vi "FPGAController_v5.vi"() -> ()   [LabVIEW 2015]
uses:
  <vilib>/Utility/miscctls.llb/LVPointTypeDef.ctl
  <vilib>/FPGAPlugInAG/PXIe-7971R/niLvFpga_Open_PXIe-7971R.vi
  <userlib>/_OpenG.lib/comparison/comparison.llb/DBL Changed__ogtk.vi
  <userlib>/_OpenG.lib/file/file.llb/Strip Path Extension - Path__ogtk.vi
  <userlib>/_OpenG.lib/comparison/comparison.llb/Boolean Changed__ogtk.vi
  <vilib>/Utility/error.llb/Error Cluster From Error Code.vi
  <vilib>/rvi/errors/niLvFpgaAdjustHostInterfaceError.vi
  <vilib>/addons/database/Connection.llb/Conn Execute.vi
  <vilib>/addons/database/Recordset.llb/Rec Fetch Recordset Data (R).vi
  <vilib>/addons/database/Recordset.llb/Rec Destroy - Connection.vi
  <vilib>/FPGAPlugInAG/PXIe-7971R/niLvFpga_Close_PXIe-7971R.vi
  <vilib>/rvi/interface/nirviOpenFPGA/nirviOpenFPGA.xnode
  FPGA Bitfiles/FPGA2_FPGATarget_FPGAcode2_Gw4Ab0yitnw.lvbitx
  <vilib>/rvi/interface/nirviMethod/nirviMethod.xnode
  <vilib>/FPGA/interface/niFpgaViExecutionMode.ctl
  <vilib>/rvi/interface/nirviReadWriteControl/nirviReadWriteControl.xnode
  <vilib>/addons/database/_DB Variant To Data/Database Variant To Data.xnode
  <vilib>/rvi/interface/nirviCloseFPGA/nirviCloseFPGA.xnode
  <vilib>/addons/database/NI_Database_API.lvlib
  NiFpgaLv.dll
panel:
  out "Time Betwee Shots":dbl
  out "Del Armed":bool
  in  "Lower Threshold":bool
  in  "Raise Threshold":bool
  out "Update Threshold":bool
  in  "Min. Time\nBetween Shots (s)":dbl
  in  "Rate Limiting":bool
  out "Armed":bool
  in  "Add Delay":bool
  in  "Delay Name":string
  in  "Delay Value":dbl=3.0 min=0.0
  in  "Delay Ring":dbl(ring)=3.15039 items=["Ablation Chamber"=6.45, "LEIL Chamber"=4.318, "Third Detector"=3.15039, "Custom"=0.0]
  in  "Rearm Trigger":bool
  in  "One Shot Mode":bool
  out "Last Update:":timestamp
  out "Updating FPGA":bool
  out "Sensitivity":dbl
  out "error out":errorcluster
  out "Low Mass Limit":fxp<+,31,17>
  out "High Mass Limit":fxp<+,31,17>
  out "stopping":bool
  in  "Auto Threshold":bool
  out "Peletron (MV)":dbl=2.0
  out "High Mass (kg)":dbl=inf
  out "Low Mass (kg)":dbl
  out "High Charge Limit":i16
  out "Low Charge Limit":i16
  out "High velocity count":i32=210
  out "Low velocity count":i32=21000
  in  "stop":bool
  in  "Peak-Threshold Factor":dbl=2.0
  out "Low Charge Limit (fC)":dbl
  out "High Charge Limit (fC)":dbl=100.0
  out "High Velocity":dbl=100000.0
  out "Low Velocity":dbl=1000.0
  out "Filter 7 Peak":i32=7483
  out "Filter 6 Peak":i32=9863
  out "Filter 5 Peak":i32=13910
  out "Filter 4 Peak":i32=18191
  out "Filter 3 Peak":i32=46254
  out "Filter 2 Peak":i32=120664
  out "Filter 1 Peak":i32=295996
  in  "Filter7 Threshold":i32=-21165
  in  "Filter6 Threshold":i32=-29358
  in  "Filter5 Threshold":i32=-41730
  in  "Filter4 Threshold":i32=-54306
  in  "Filter3 Threshold":i32=-138762
  in  "Filter2 Threshold":i32=-361992
  in  "Filter1 Threshold":i32=-887988
  in  "Zero Peak Values":bool
  in  "Assign Threshold":bool
  in  "Run Mode":bool
  # "Settings"
  # "Dubugging"
  # "Independent Variable"
  # "Low Vel."
  # "High Vel."
  # "Low Q (fC)"
  # "High Q (fC)"
  # "Plate Control While Loop Counter"
  # "Low Mass (kg)"
  # "High Mass (kg)"
  # "Sens. (V/pC)"
  # "Peletron (MV)"
  # "Current Value of Running Average"
  # "Peak Threshold Factor"
  # "Delay Trigger"
  # "Dist. from 2nd Det. (m)"
  # "Name"
  # "Peak Values"
  # "Peak 1"
  # "Peak 2"
  # "Peak 3"
  # "Peak 4"
  # "Peak 5"
  # "Peak 6"
  # "Peak 7"
  # "Thresholds"
  # "Threshold 1"
  # "Threshold 2"
  # "Threshold 3"
  # "Threshold 4"
  # "Threshold 5"
  # "Threshold 6"
  # "Threshold 7"
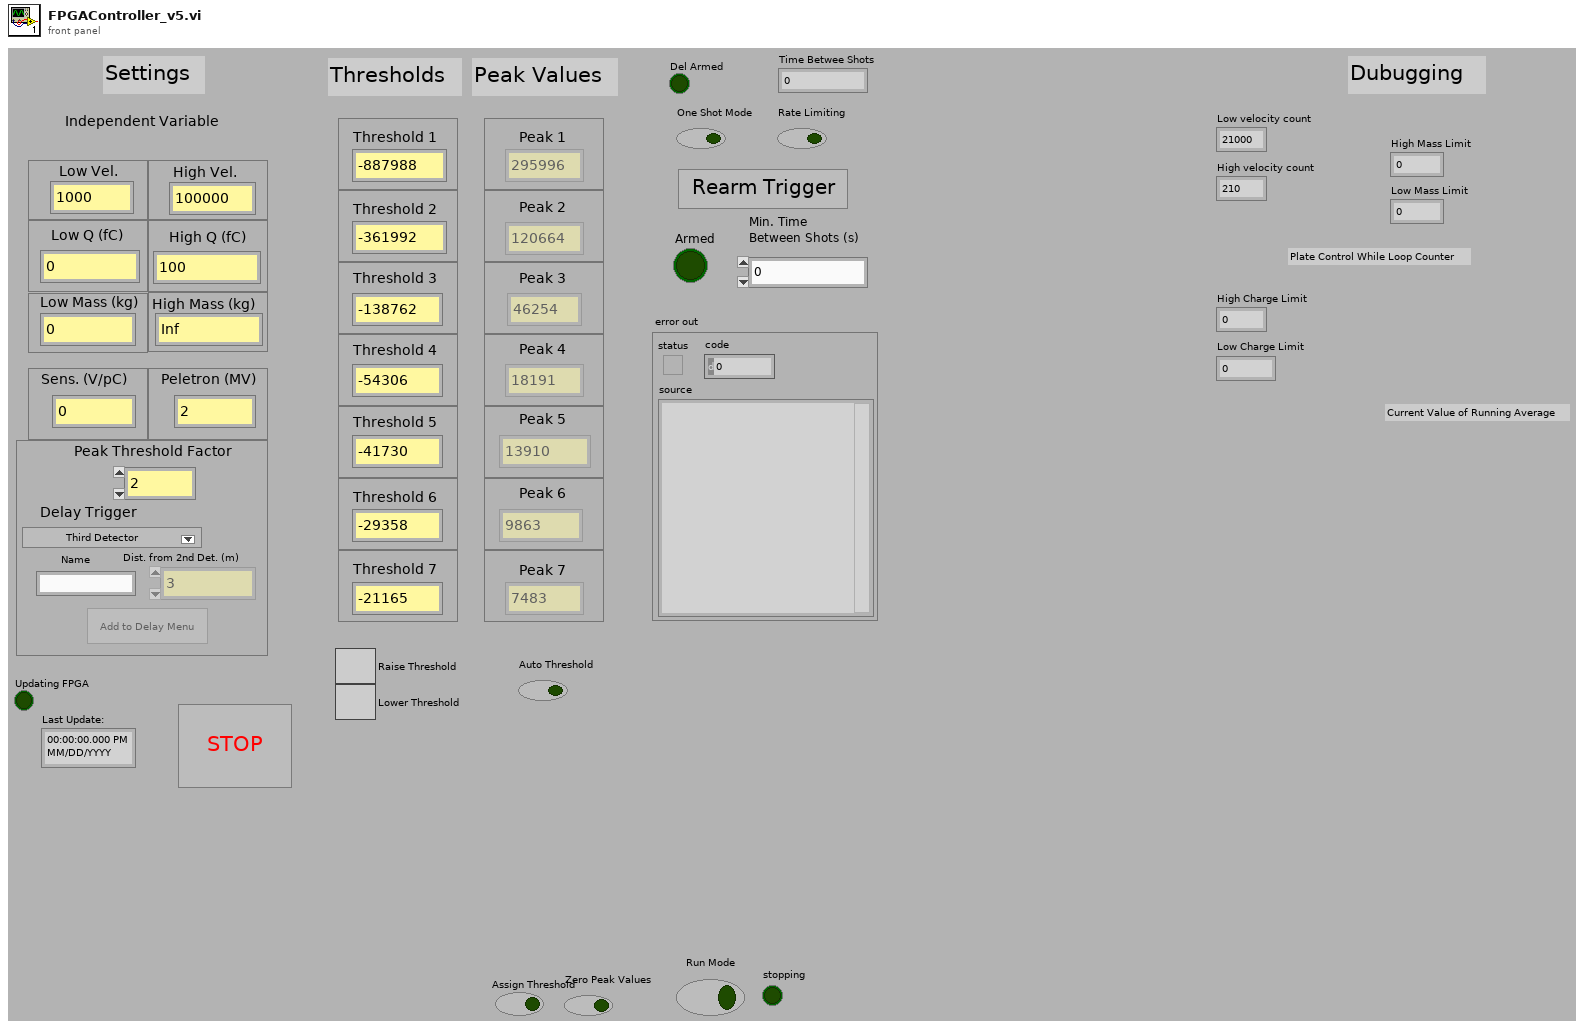
[diagram p1: front panel]
types:
  T1 = typedef "LVPointTypeDef.ctl" = cluster{"Horizontal":i16, "Vertical":i16}
  T2 = enum8{"Enabled", "Disabled", "Disabled and Grayed Out"}
  T3 = typedef "NI_Database_API.lvlib/Conn ObjectReference.ctl" = refnum<k1>
  T4 = cluster{"Filter 1 Peak":i32, "Filter 2 Peak":i32, "Filter 3 Peak":i32, "Filter 4 Peak":i32, "Filter 5 Peak":i32, "Filter 6 Peak":i32, "Filter 7 Peak":i32}
  T5 = typedef "NI_Database_API.lvlib/Rec ObjectReference.ctl" = refnum<k1>
  T6 = cluster{"Numeric":dbl, "Numeric":dbl, "Numeric":dbl, "Numeric":dbl, "Numeric":dbl, "Numeric":dbl, dbl, dbl, "Value":dbl, fxp<+,16,7>, bool}
  T7 = typedef "LVStringsAndValuesArrayTypeDef_DBL.ctl" = cluster{"String":string, "Value":dbl}[]
  T8 = cluster{"Low Velocity Count":i32, "High Velocity Count":i32, "Low Charge Limit (ADC ticks)":i16, "High Charge Limit (ADC ticks)":i16, "Low Mass (ADC*cycle^2)":i64, "High Mass (ADC*cycle^2)":i64, "Mult":fxp<+,16,7>, "Mult Use?":bool}
  T9 = cluster{"Detector 3 Correlation 1":i16, "Detector 3 Correlation 2":i16, "Detector 3 Correlation 3":i16, "Detector 3 Correlation 4":i16, "Detector 3 Correlation 5":i16, "Detector 3 Correlation 6":i16, "Detector 3 Correlation 7":i16}
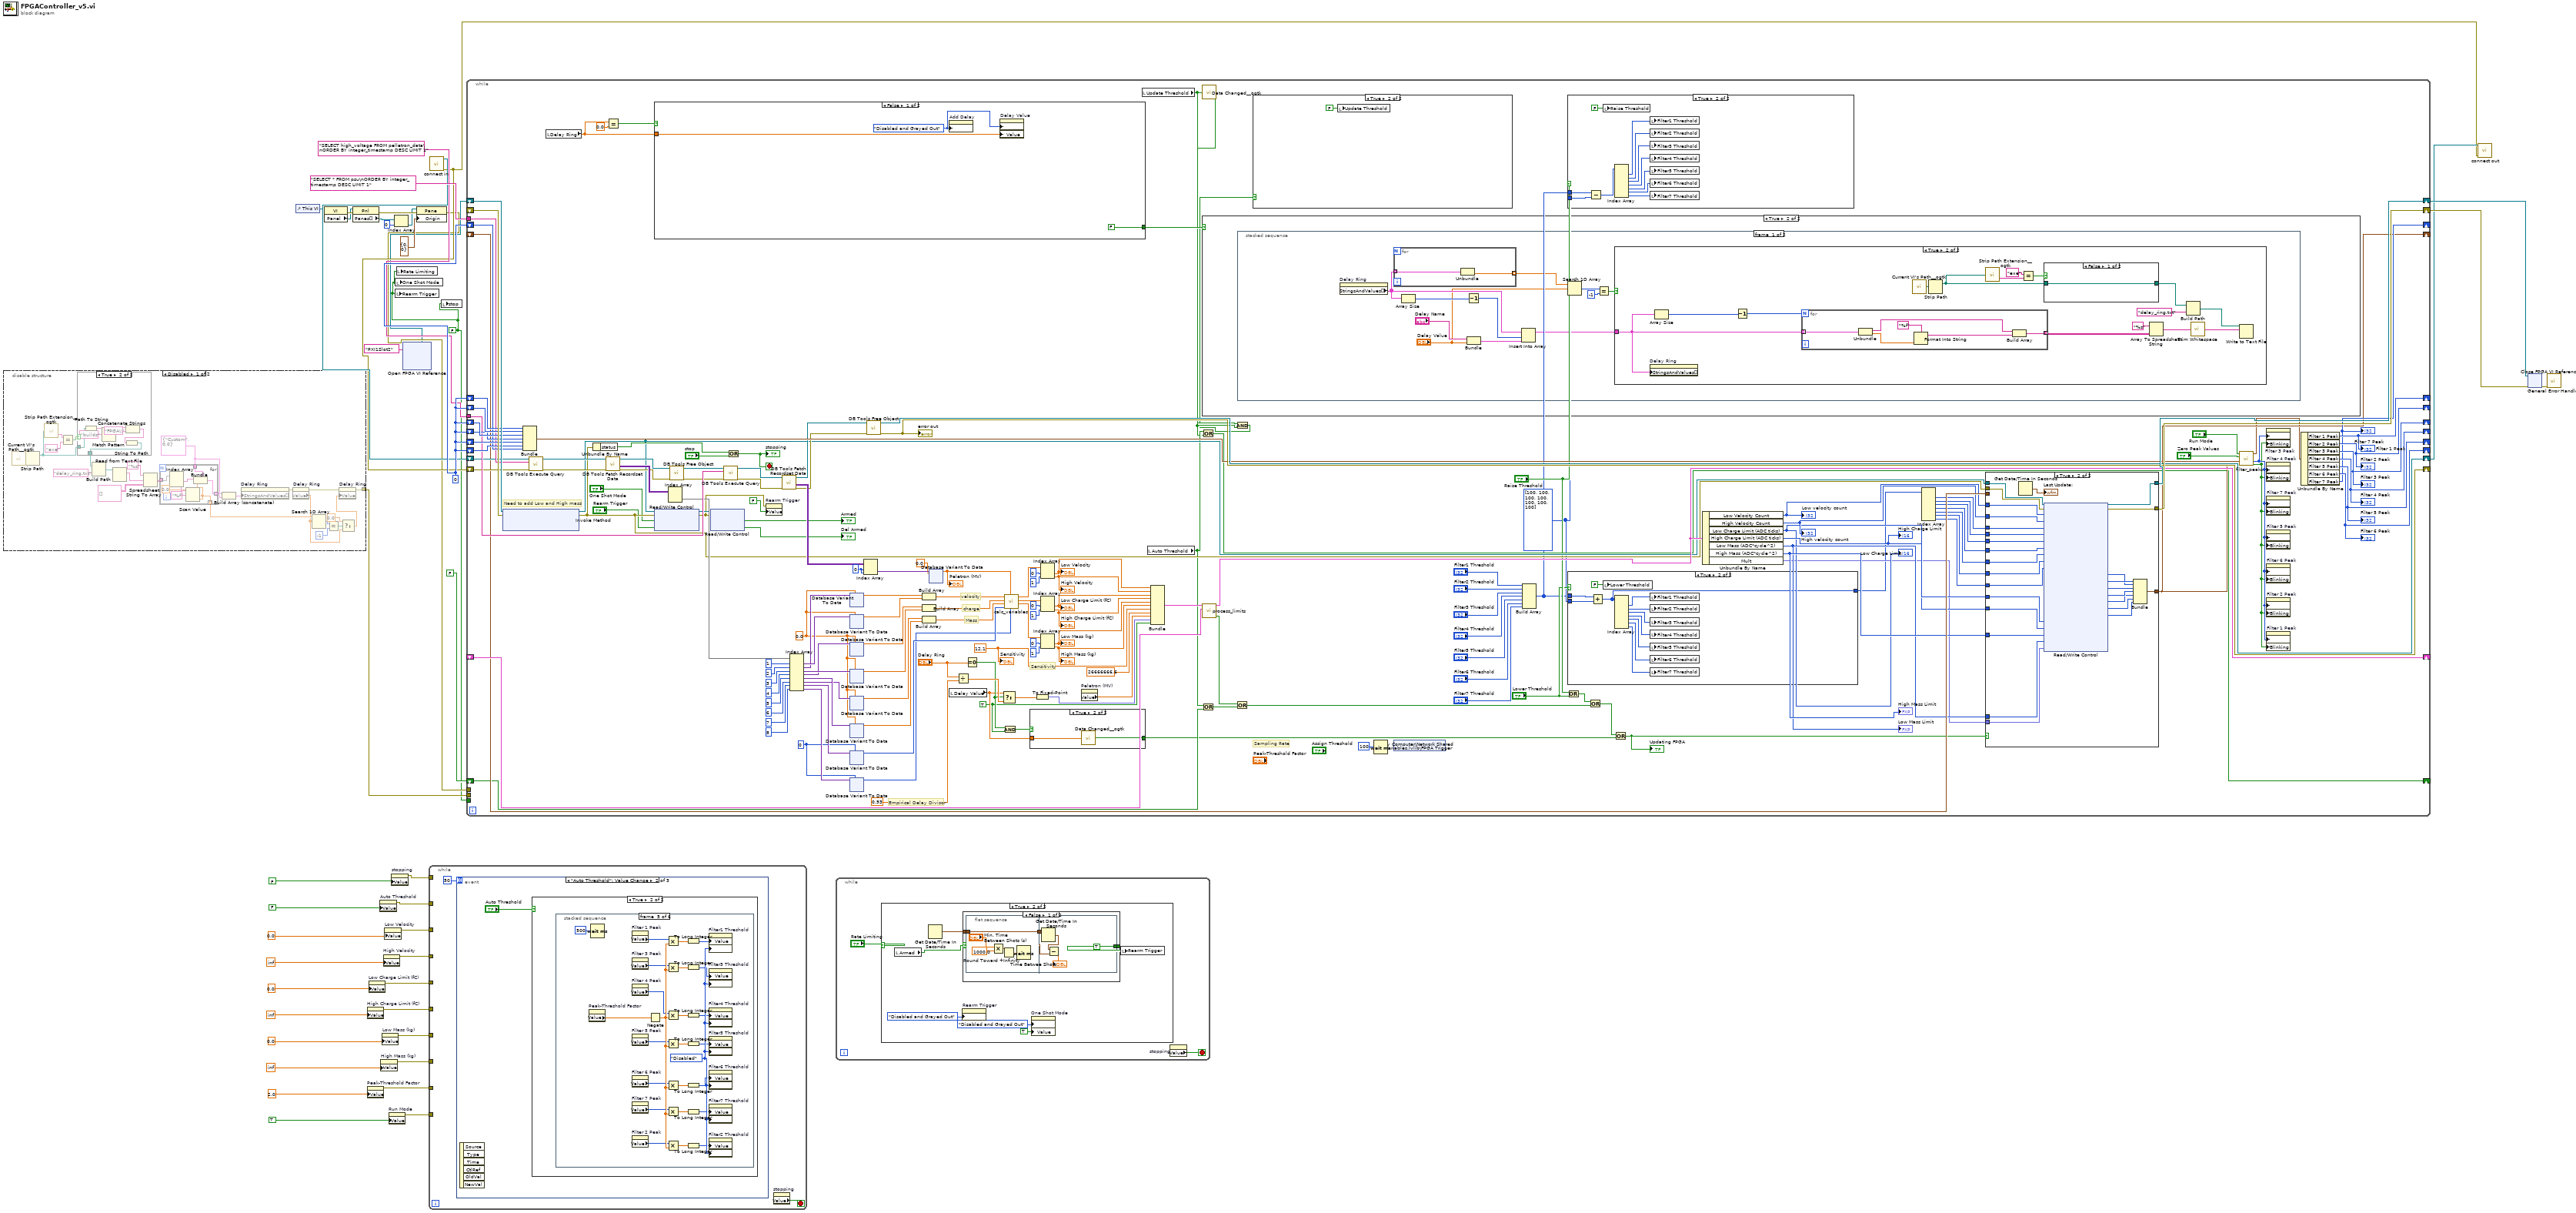
[diagram p0: block diagram]
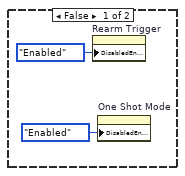
[diagram p4: hidden frame]
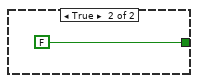
[diagram p5: hidden frame]
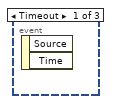
[diagram p6: hidden frame]
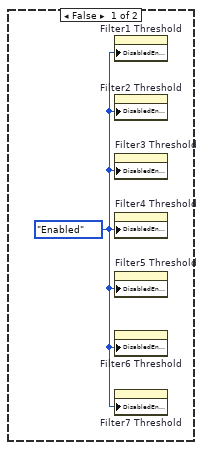
[diagram p7: hidden frame]
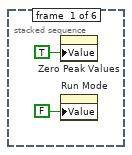
[diagram p8: hidden frame]
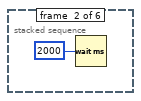
[diagram p9: hidden frame]
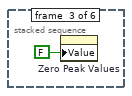
[diagram p10: hidden frame]
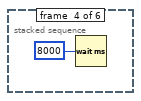
[diagram p11: hidden frame]
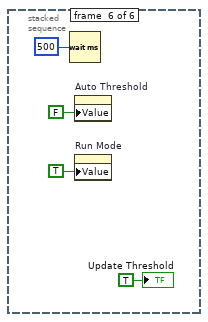
[diagram p12: hidden frame]
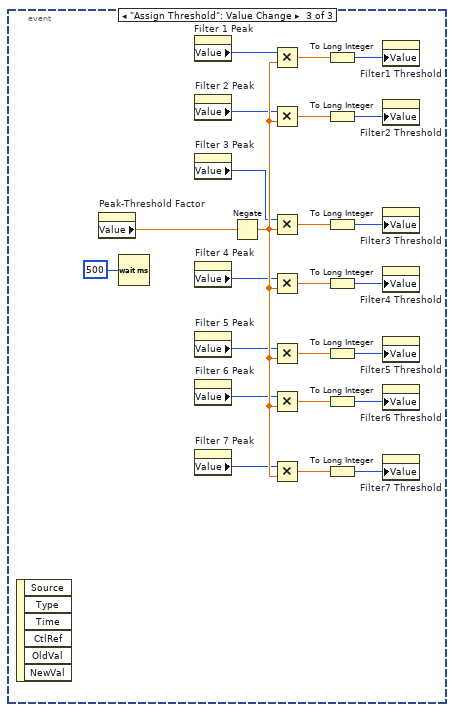
[diagram p13: hidden frame]
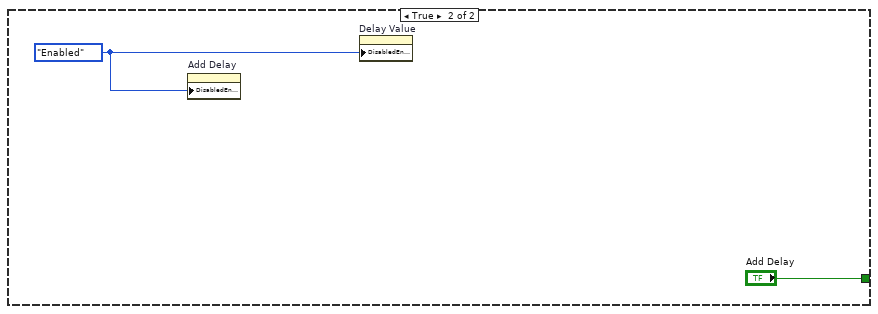
[diagram p18: hidden frame]
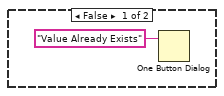
[diagram p20: hidden frame]
diagram:
  w1 = FALSE
  w42 = 0
  n1 = disable-structure shown="Disabled" {
    disable-tunnel: [w50 _] -> w3
    frame Disabled {
      w59 = cluster{"String":string, "Value":dbl} {"String"="Custom", "Value"=0.0}
      n2 = call <userlib>:"Current VI's Path__ogtk.vi"() -> ("Current VI's Path (+ Relative)"=w68:path)  [unwired: 1 in]
      n3 = Strip Path(path=w68) -> (stripped path=w54:path)  [unwired: 1 out]
      n4 = call-poly <userlib>:"Strip Path Extension__ogtk.vi"("path"=w54) -> ("extension"=w58:string)  [unwired: 1 out]
      n5 = Equal?(x=w58, y="exe") -> (x = y?=w55:bool)
      n6 = case shown="True" w55 {
        tunnel: w54 -> [w77 w84]
        tunnel: [w77 w78] -> w53
        frame False {
        }
        frame True {
          n7 = Path To String(path=w84) -> (string=w83:string)
          n8 = Match Pattern(string=w83, regular expression="builds") -> (before substring=w81:string)  [unwired: 1 in, 3 out]
          n9 = Concatenate Strings(w81, "FPGA\\" ("string")) -> (w79:string)
          n10 = String To Path(string=w79) -> (path=w78:path)
        }
      }
      n11 = Build Path(base path=w53, name or relative path="delay_ring.txt") -> (appended path=w56:path)
      n12 = Read from Text File(file (use dialog)=w56) -> (text=w66:string)  [unwired: 3 in, 3 out]
      n13 = Spreadsheet String To Array(format string="%s", spreadsheet string=w66, array type (2D Dbl)=string[][] []) -> (array=w63:string[][])  [unwired: 1 in]
      n14 = for {
        tunnel: w63 -> [w76] mode=indexing
        tunnel: w59 -> [w74]
        tunnel: [w70] -> w60 mode=indexing
        tunnel: [w69] -> w52 mode=indexing
        n15 = Index Array(array=w76) -> (element #1=w75:string, element #2=w73:string)  [unwired: 2 in]
        n16 = Scan Value(string=w73, format string="%f", default (0 dbl)=0.0) -> (value=w69:dbl)  [unwired: 1 out]
        n17 = Bundle(cluster=w74, "String"=w75, "Value"=w69) -> (w70:cluster{"String":string, "Value":dbl})
      }
      n18 = Build Array (concatenate)(w60, w59) -> (w62:cluster{"String":string, "Value":dbl}[])
      n19 = property on="Delay Ring" class="Ring (strict)"("StringsAndValues[]"=w62) -> (error out=w61:errorcluster)  [unwired: 2 in, 1 out]
      n20 = property on="Delay Ring" class="Ring (strict)"(error in=w61) -> (error out=w51:errorcluster, "Value"=w45:dbl)  [unwired: 1 in, 1 out]
      n21 = Search 1D Array(1D array=w52, element=w45) -> (index of element=w49:i32)  [unwired: 1 in]
      n22 = Equal?(x=w49, y=-1) -> (x = y?=w47:bool)
      n23 = Select(t=0.0, s=w47, f=w45) -> (s? t:f=w46:dbl)
      n24 = property on="Delay Ring" class="Ring (strict)"(error in=w51, "Value"=w46) -> (error out=w50:errorcluster)  [unwired: 1 in, 1 out]
    }
    frame Enabled {
    }
  }
  n25 = control-ref of="This VI"() -> (w14:refnum<vi>)
  n26 = property class="VI"(reference=w14) -> (error out=w13:errorcluster, "Panel"=w12:refnum<vi>)  [unwired: 1 in, 1 out]
  n27 = property class="Pnl"(reference=w12, error in=w13) -> (error out=w11:errorcluster, "Panes[]"=w10:refnum<vi>[])  [unwired: 1 out]
  n28 = property on="High Charge Limit (fC)" class="DigNum (strict)"("Value"=inf ("High Charge Limit (fC)")) -> (error out=w29:errorcluster)  [unwired: 2 in, 1 out]
  n29 = property on="Peak-Threshold Factor" class="DigNum (strict)"("Value"=2.0 ("Peak-Threshold Factor")) -> (error out=w23:errorcluster)  [unwired: 2 in, 1 out]
  n30 = property on="Low Charge Limit (fC)" class="DigNum (strict)"("Value"=0.0 ("Low Charge Limit (fC)")) -> (error out=w31:errorcluster)  [unwired: 2 in, 1 out]
  n31 = property on="Auto Threshold" class="Bool (strict)"("Value"=FALSE ("Auto Threshold")) -> (error out=w37:errorcluster)  [unwired: 2 in, 1 out]
  n32 = property on="High Mass (kg)" class="DigNum (strict)"("Value"=inf ("High Mass (kg)")) -> (error out=w25:errorcluster)  [unwired: 2 in, 1 out]
  n33 = property on="Low Mass (kg)" class="DigNum (strict)"("Value"=0.0 ("Low Mass (kg)")) -> (error out=w27:errorcluster)  [unwired: 2 in, 1 out]
  n34 = property on="High Velocity" class="DigNum (strict)"("Value"=inf ("High Velocity")) -> (error out=w33:errorcluster)  [unwired: 2 in, 1 out]
  n35 = property on="Low Velocity" class="DigNum (strict)"("Value"=0.0 ("Low Velocity")) -> (error out=w35:errorcluster)  [unwired: 2 in, 1 out]
  n36 = property on="Run Mode" class="Bool (strict)"("Value"=TRUE ("Run Mode")) -> (error out=w21:errorcluster)  [unwired: 2 in, 1 out]
  n37 = property on="stopping" class="Bool (strict)"("Value"=FALSE ("stopping")) -> (error out=w39:errorcluster)  [unwired: 2 in, 1 out]
  n38 = Index Array(array=w10, index=0) -> (element=w8:refnum<vi>)
  n39 = local write "Rearm Trigger"(w1) -> ()
  n40 = local write "One Shot Mode"(w1) -> ()
  n41 = local write "Rate Limiting"(w1) -> ()
  n42 = xnode "Open FPGA VI Reference"("resource name"=tag "PXI1Slot2") -> ("FPGA VI Reference Out"=w5:refnum<k20>)  [unwired: 1 in, 1 out]
  n43 = property class="Pane"(reference=w8, error in=w11, "Origin"=T1 {"Horizontal"=0, "Vertical"=0}) -> (error out=w6:errorcluster)  [unwired: 1 out]
  n44 = while {
    tunnel: w39 -> [_]
    tunnel: w37 -> [_]
    tunnel: w35 -> [_]
    tunnel: w33 -> [_]
    tunnel: w31 -> [_]
    tunnel: w29 -> [_]
    tunnel: w27 -> [_]
    tunnel: w25 -> [_]
    tunnel: w23 -> [_]
    tunnel: w21 -> [_]
    stop <- w86 stop-if-true
    n45 = event shown="[1] \"Auto Threshold\": Value Change" {
      selector: _ -> [_ _ _]
      dyn-events: _ -> [_ _ _]
      timeout: 50 -> [_ _ _]
      event Timeout {
        n46 = event-data() -> ()  [unwired: 1 in, 2 out]
      }
      event "Auto Threshold": Value Change {
        n47 = event-data() -> ()  [unwired: 1 in, 6 out]
        n48 = case shown="True" "Auto Threshold" {
          frame False {
            w88 = T2."Enabled" ("Disabled")
            n49 = property on="Filter1 Threshold" class="DigNum (strict)"("DisabledEnum"=w88) -> ()  [unwired: 2 in, 2 out]
            n50 = property on="Filter2 Threshold" class="DigNum (strict)"("DisabledEnum"=w88) -> ()  [unwired: 2 in, 2 out]
            n51 = property on="Filter3 Threshold" class="DigNum (strict)"("DisabledEnum"=w88) -> ()  [unwired: 2 in, 2 out]
            n52 = property on="Filter4 Threshold" class="DigNum (strict)"("DisabledEnum"=w88) -> ()  [unwired: 2 in, 2 out]
            n53 = property on="Filter5 Threshold" class="DigNum (strict)"("DisabledEnum"=w88) -> ()  [unwired: 2 in, 2 out]
            n54 = property on="Filter6 Threshold" class="DigNum (strict)"("DisabledEnum"=w88) -> ()  [unwired: 2 in, 2 out]
            n55 = property on="Filter7 Threshold" class="DigNum (strict)"("DisabledEnum"=w88) -> ()  [unwired: 2 in, 2 out]
          }
          frame True {
            n56 = stacked-sequence {
              frame #0 {
                n57 = property on="Zero Peak Values" class="Bool (strict)"("Value"=TRUE ("Zero Peak Values")) -> ()  [unwired: 2 in, 2 out]
                n58 = property on="Run Mode" class="Bool (strict)"("Value"=FALSE ("Run Mode")) -> ()  [unwired: 2 in, 2 out]
              }
              frame #1 {
                n59 = Wait (ms)(milliseconds to wait=u32 2000) -> ()  [unwired: 1 out]
              }
              frame #2 {
                n60 = property on="Zero Peak Values" class="Bool (strict)"("Value"=FALSE ("Zero Peak Values")) -> ()  [unwired: 2 in, 2 out]
              }
              frame #3 {
                n61 = Wait (ms)(milliseconds to wait=u32 8000) -> ()  [unwired: 1 out]
              }
              frame #4 {
                w118 = T2."Disabled" ("Disabled")
                n62 = property on="Peak-Threshold Factor" class="DigNum (strict)"() -> ("Value"=w103:dbl)  [unwired: 2 in, 2 out]
                n63 = Wait (ms)(milliseconds to wait=u32 500) -> ()  [unwired: 1 out]
                n64 = property on="Filter 1 Peak" class="DigNum (strict)"() -> ("Value"=w101:i32)  [unwired: 2 in, 2 out]
                n65 = property on="Filter 3 Peak" class="DigNum (strict)"() -> ("Value"=w99:i32)  [unwired: 2 in, 2 out]
                n66 = property on="Filter 4 Peak" class="DigNum (strict)"() -> ("Value"=w98:i32)  [unwired: 2 in, 2 out]
                n67 = property on="Filter 5 Peak" class="DigNum (strict)"() -> ("Value"=w97:i32)  [unwired: 2 in, 2 out]
                n68 = property on="Filter 6 Peak" class="DigNum (strict)"() -> ("Value"=w96:i32)  [unwired: 2 in, 2 out]
                n69 = property on="Filter 7 Peak" class="DigNum (strict)"() -> ("Value"=w95:i32)  [unwired: 2 in, 2 out]
                n70 = property on="Filter 2 Peak" class="DigNum (strict)"() -> ("Value"=w100:i32)  [unwired: 2 in, 2 out]
                n71 = Negate(x=w103) -> (-x=w102:dbl)
                n72 = Multiply(x=w101, y=w102) -> (x*y=w117:dbl)
                n73 = Multiply(x=w99, y=w102) -> (x*y=w113:dbl)
                n74 = Multiply(x=w98, y=w102) -> (x*y=w111:dbl)
                n75 = Multiply(x=w97, y=w102) -> (x*y=w109:dbl)
                n76 = Multiply(x=w96, y=w102) -> (x*y=w107:dbl)
                n77 = Multiply(x=w95, y=w102) -> (x*y=w105:dbl)
                n78 = Multiply(x=w100, y=w102) -> (x*y=w115:dbl)
                n79 = To Long Integer(number=w117) -> (32bit integer=w116:i32)
                n80 = To Long Integer(number=w113) -> (32bit integer=w112:i32)
                n81 = To Long Integer(number=w111) -> (32bit integer=w110:i32)
                n82 = To Long Integer(number=w109) -> (32bit integer=w108:i32)
                n83 = To Long Integer(number=w107) -> (32bit integer=w106:i32)
                n84 = To Long Integer(number=w105) -> (32bit integer=w104:i32)
                n85 = To Long Integer(number=w115) -> (32bit integer=w114:i32)
                n86 = property on="Filter1 Threshold" class="DigNum (strict)"("Value"=w116, "DisabledEnum"=w118) -> ()  [unwired: 2 in, 2 out]
                n87 = property on="Filter3 Threshold" class="DigNum (strict)"("Value"=w112, "DisabledEnum"=w118) -> ()  [unwired: 2 in, 2 out]
                n88 = property on="Filter4 Threshold" class="DigNum (strict)"("Value"=w110, "DisabledEnum"=w118) -> ()  [unwired: 2 in, 2 out]
                n89 = property on="Filter5 Threshold" class="DigNum (strict)"("Value"=w108, "DisabledEnum"=w118) -> ()  [unwired: 2 in, 2 out]
                n90 = property on="Filter6 Threshold" class="DigNum (strict)"("Value"=w106, "DisabledEnum"=w118) -> ()  [unwired: 2 in, 2 out]
                n91 = property on="Filter7 Threshold" class="DigNum (strict)"("Value"=w104, "DisabledEnum"=w118) -> ()  [unwired: 2 in, 2 out]
                n92 = property on="Filter2 Threshold" class="DigNum (strict)"("Value"=w114, "DisabledEnum"=w118) -> ()  [unwired: 2 in, 2 out]
              }
              frame #5 {
                n93 = Wait (ms)(milliseconds to wait=u32 500) -> ()  [unwired: 1 out]
                n94 = property on="Auto Threshold" class="Bool (strict)"("Value"=FALSE ("Auto Threshold")) -> ()  [unwired: 2 in, 2 out]
                n95 = property on="Run Mode" class="Bool (strict)"("Value"=TRUE ("Run Mode")) -> ()  [unwired: 2 in, 2 out]
                "Update Threshold" <- TRUE ("Update Threshold")
              }
            }
          }
        }
      }
      event "Assign Threshold": Value Change {
        n96 = event-data() -> ()  [unwired: 1 in, 6 out]
        n97 = property on="Peak-Threshold Factor" class="DigNum (strict)"() -> ("Value"=w137:dbl)  [unwired: 2 in, 2 out]
        n98 = Wait (ms)(milliseconds to wait=u32 500) -> ()  [unwired: 1 out]
        n99 = property on="Filter 1 Peak" class="DigNum (strict)"() -> ("Value"=w136:i32)  [unwired: 2 in, 2 out]
        n100 = property on="Filter 2 Peak" class="DigNum (strict)"() -> ("Value"=w135:i32)  [unwired: 2 in, 2 out]
        n101 = property on="Filter 3 Peak" class="DigNum (strict)"() -> ("Value"=w134:i32)  [unwired: 2 in, 2 out]
        n102 = property on="Filter 4 Peak" class="DigNum (strict)"() -> ("Value"=w133:i32)  [unwired: 2 in, 2 out]
        n103 = property on="Filter 5 Peak" class="DigNum (strict)"() -> ("Value"=w132:i32)  [unwired: 2 in, 2 out]
        n104 = property on="Filter 6 Peak" class="DigNum (strict)"() -> ("Value"=w131:i32)  [unwired: 2 in, 2 out]
        n105 = property on="Filter 7 Peak" class="DigNum (strict)"() -> ("Value"=w130:i32)  [unwired: 2 in, 2 out]
        n106 = Negate(x=w137) -> (-x=w139:dbl)
        n107 = Multiply(x=w136, y=w139) -> (x*y=w146:dbl)
        n108 = Multiply(x=w135, y=w139) -> (x*y=w144:dbl)
        n109 = Multiply(x=w134, y=w139) -> (x*y=w143:dbl)
        n110 = Multiply(x=w133, y=w139) -> (x*y=w142:dbl)
        n111 = Multiply(x=w132, y=w139) -> (x*y=w141:dbl)
        n112 = Multiply(x=w131, y=w139) -> (x*y=w140:dbl)
        n113 = Multiply(x=w130, y=w139) -> (x*y=w145:dbl)
        n114 = To Long Integer(number=w146) -> (32bit integer=w129:i32)
        n115 = To Long Integer(number=w144) -> (32bit integer=w128:i32)
        n116 = To Long Integer(number=w143) -> (32bit integer=w127:i32)
        n117 = To Long Integer(number=w142) -> (32bit integer=w126:i32)
        n118 = To Long Integer(number=w141) -> (32bit integer=w125:i32)
        n119 = To Long Integer(number=w140) -> (32bit integer=w124:i32)
        n120 = To Long Integer(number=w145) -> (32bit integer=w123:i32)
        n121 = property on="Filter1 Threshold" class="DigNum (strict)"("Value"=w129) -> ()  [unwired: 2 in, 2 out]
        n122 = property on="Filter2 Threshold" class="DigNum (strict)"("Value"=w128) -> ()  [unwired: 2 in, 2 out]
        n123 = property on="Filter3 Threshold" class="DigNum (strict)"("Value"=w127) -> ()  [unwired: 2 in, 2 out]
        n124 = property on="Filter4 Threshold" class="DigNum (strict)"("Value"=w126) -> ()  [unwired: 2 in, 2 out]
        n125 = property on="Filter5 Threshold" class="DigNum (strict)"("Value"=w125) -> ()  [unwired: 2 in, 2 out]
        n126 = property on="Filter6 Threshold" class="DigNum (strict)"("Value"=w124) -> ()  [unwired: 2 in, 2 out]
        n127 = property on="Filter7 Threshold" class="DigNum (strict)"("Value"=w123) -> ()  [unwired: 2 in, 2 out]
      }
    }
    n128 = property on="stopping" class="Bool (strict)"() -> ("Value"=w86:bool)  [unwired: 2 in, 2 out]
  }
  n129 = call "connect in.vi"() -> ("error out"=w15:errorcluster, "Database Connection"=w16:T3)  [unwired: 7 in, 1 out]
  n130 = local write "stop"(w1) -> ()
  n131 = while {
    shift-right: [w306] -> w41
    shift-left: w5 -> [w310]
    shift-right: [w305] -> w40
    shift-left: _ -> [w309]
    shift-right: [w301] -> _
    shift-left: w42 -> [w294]
    shift-right: [w300] -> _
    shift-left: w42 -> [w293]
    shift-right: [w299] -> _
    shift-left: w42 -> [w292]
    shift-right: [w298] -> _
    shift-left: w42 -> [w291]
    shift-right: [w297] -> _
    shift-left: w42 -> [w290]
    shift-right: [w303] -> _
    shift-left: w42 -> [w296]
    shift-right: [w302] -> _
    shift-left: w42 -> [w295]
    tunnel: "SELECT * FROM psu\nORDER BY integer_timestamp DESC LIMIT 1" ("SQL query") -> [w289]
    tunnel: "SELECT high_voltage FROM pelletron_data\nORDER BY integer_timestamp DESC LIMIT 1" ("SQL query") -> [w288]
    shift-right: [w284] -> w17
    shift-left: w16 -> [w287]
    shift-right: [w285] -> _
    shift-left: w15 -> [w286]
    shift-right: [w283] -> _
    shift-left: _ -> [w282]
    shift-right: [w280] -> _
    shift-left: _ -> [w281]
    tunnel: w6 -> [_]
    tunnel: w3 -> [_]
    shift-right: [w186] -> _
    shift-left: FALSE -> [w189]
    tunnel: w1 -> [_]
    stop <- w304 stop-if-true
    w150 = i32[] [100, 100, 100, 100, 100, 100, 100]
    w151 = TRUE
    w236 = 0 ("index (row)")
    w244 = i8 0
    w245 = 0.0
    w210 = 12.1
    # "charge"
    # "Empirical Delay Divisor"
    # "Mass"
    # "velocity"
    # "Sensitivity"
    # "Sampling Rate"
    # "Need to add Low and High mass"
    n132 = xnode "Invoke Method"("FPGA VI Reference In"=w310, "error in"=w309) -> ("FPGA VI Reference Out"=w204:refnum<k20>, "error out"=w203:errorcluster)  [unwired: 1 out]
    n133 = Bundle("Filter 1 Peak"=w296, "Filter 2 Peak"=w295, "Filter 3 Peak"=w294, "Filter 4 Peak"=w293, "Filter 5 Peak"=w292, "Filter 6 Peak"=w291, "Filter 7 Peak"=w290) -> (w276:T4)  [unwired: 1 in]
    n134 = call-poly <vilib>:"DB Tools Execute Query.vi"("error in (no error)"=w286, "SQL query"=w289, "connection reference"=w287) -> ("error out"=w264:errorcluster, "recordset reference"=w265:T5)  [unwired: 5 in]
    n135 = local read "Delay Ring"() -> (w190:dbl)
    n136 = Unbundle By Name(w203) -> ("status"=w308:bool)
    n137 = call-poly <vilib>:"DB Tools Fetch Recordset Data.vi"("error in (no error)"=w264, "recordset reference"=w265) -> ("error out"=w242:errorcluster, "recordset data"=w255:variant[][], "recordset reference out"=w243:T5)  [unwired: 3 in]
    n138 = Equal?(x=w190, y=0.0) -> (x = y?=w191:bool)
    n139 = case shown="False" w191 {
      tunnel: [FALSE ("Add Delay") "Add Delay"] -> w207
      tunnel: w190 -> [w339 _]
      frame False {
        w340 = T2."Disabled and Grayed Out" ("Disabled")
        n140 = property on="Add Delay" class="Bool (strict)"("DisabledEnum"=w340) -> ()  [unwired: 2 in, 2 out]
        n141 = property on="Delay Value" class="DigNum (strict)"("DisabledEnum"=w340, "Value"=w339) -> ()  [unwired: 2 in, 2 out]
      }
      frame True {
        w341 = T2."Enabled" ("Disabled")
        n142 = property on="Add Delay" class="Bool (strict)"("DisabledEnum"=w341) -> ()  [unwired: 2 in, 2 out]
        n143 = property on="Delay Value" class="DigNum (strict)"("DisabledEnum"=w341) -> ()  [unwired: 2 in, 2 out]
      }
    }
    n144 = xnode "Read/Write Control"("FPGA VI Reference In"=w204, "error in"=w203, "One Shot"="One Shot Mode", "Reset One Shot"="Rearm Trigger") -> ("FPGA VI Reference Out"=w198:refnum<k20>, "error out"=w197:errorcluster)
    n145 = Index Array(array=w255) -> (element=w254:variant[])  [unwired: 2 in]
    n146 = call-poly <vilib>:"DB Tools Free Object.vi"("error in (no error)"=w242, "recordset reference"=w243) -> ("error out"=w240:errorcluster, "connection reference"=w241:T3)  [unwired: 8 in]
    n147 = xnode "Read/Write Control"("FPGA VI Reference In"=w198, "error in"=w197) -> ("Armed"=→"Armed":bool, "Del Armed"=→"Del Armed":bool)  [unwired: 2 out]
    n148 = call-poly <vilib>:"DB Tools Execute Query.vi"("error in (no error)"=w240, "SQL query"=w288, "connection reference"=w241) -> ("error out"=w238:errorcluster, "recordset reference"=w239:T5)  [unwired: 5 in]
    n149 = Or(x=w308, y="stop") -> (x .or. y?=w304:bool)
    "stopping" <- w304
    n150 = property on="Rearm Trigger" class="Bool (strict)"(error in=w197, "Value"=FALSE ("Rearm Trigger")) -> ()  [unwired: 1 in, 2 out]
    n151 = call-poly <vilib>:"DB Tools Fetch Recordset Data.vi"("error in (no error)"=w238, "recordset reference"=w239) -> ("error out"=w211:errorcluster, "recordset data"=w237:variant[][], "recordset reference out"=w212:T5)  [unwired: 3 in]
    n152 = Index Array(array=w254, index #1=1 ("index"), index #2=2 ("index"), index #3=3 ("index"), index #4=4 ("index"), index #5=5 ("index"), index #6=6 ("index"), index #7=7 ("index"), index #8=8 ("index")) -> (element #1=w253:variant, element #2=w252:variant, element #3=w251:variant, element #4=w250:variant, element #5=w249:variant, element #6=w248:variant, element #7=w247:variant, element #8=w246:variant)
    n153 = xnode "Database Variant To Data"("database variant"=w252, "type"=w245) -> ("data"=w162:dbl)  [unwired: 1 in, 1 out]
    n154 = xnode "Database Variant To Data"("database variant"=w253, "type"=w245) -> ("data"=w163:dbl)  [unwired: 1 in, 1 out]
    n155 = xnode "Database Variant To Data"("database variant"=w250, "type"=w245) -> ("data"=w161:dbl)  [unwired: 1 in, 1 out]
    n156 = xnode "Database Variant To Data"("database variant"=w251, "type"=w245) -> ("data"=w160:dbl)  [unwired: 1 in, 1 out]
    n157 = xnode "Database Variant To Data"("database variant"=w248, "type"=w245) -> ("data"=w159:dbl)  [unwired: 1 in, 1 out]
    n158 = xnode "Database Variant To Data"("database variant"=w249, "type"=w245) -> ("data"=w158:dbl)  [unwired: 1 in, 1 out]
    n159 = xnode "Database Variant To Data"("database variant"=w247, "type"=w244) -> ("data"=w229:i8)  [unwired: 1 in, 1 out]
    n160 = xnode "Database Variant To Data"("database variant"=w246, "type"=w244) -> ("data"=w228:i8)  [unwired: 1 in, 1 out]
    n161 = Index Array(array=w237, index (row)=w236, index (col)=w236) -> (element=w235:variant)
    n162 = call-poly <vilib>:"DB Tools Free Object.vi"("error in (no error)"=w211, "recordset reference"=w212) -> ("error out"=w285:errorcluster, "connection reference"=w284:T3)  [unwired: 8 in]
    "error out" <- w285
    n163 = Build Array(w162, w163) -> (w232:dbl[])
    n164 = Build Array(w161, w160) -> (w231:dbl[])
    n165 = Build Array(w159, w158) -> (w230:dbl[])
    n166 = xnode "Database Variant To Data"("database variant"=w235, "type"=0.0) -> ("data"=w157:dbl)  [unwired: 1 in, 1 out]
    "Peletron (MV)" <- w157
    n167 = local read "Delay Value"() -> (w155:dbl)
    n168 = Divide(x="Delay Ring", y=0.93) -> (x/y=w195:dbl)
    n169 = Equal To 0?(x="Delay Ring") -> (x = 0?=w156:bool)
    n170 = Select(t=w155, s=w156, f=w195) -> (s? t:f=w194:dbl)
    n171 = And(x=w156, y=w151) -> (x .and. y?=w152:bool)
    n172 = call "calc_variables.vi"("var2"=w228, "Peletron"=w157, "var1"=w229, "Mass"=w230, "Charge"=w231, "Velocity"=w232) -> ("Mass out"=w221:dbl[], "Charge out"=w224:dbl[], "Velocity out"=w227:dbl[])  [unwired: 3 in]
    n173 = case shown="True" w152 {
      selector: w152 -> [w311 _]
      tunnel: w155 -> [_ w313]
      tunnel: [w311 w312] -> w153
      frame False {
      }
      frame True {
        n174 = call-poly <userlib>:"Data Changed__ogtk.vi"("DBL"=w313) -> ("Changed"=w312:bool)
      }
    }
    n175 = To Fixed-Point(number=w194) -> (fixed-point=w206:fxp<+,16,7>)  [unwired: 1 in]
    n176 = Index Array(array=w227, index #1=0 ("index"), index #2=1 ("index")) -> (element #1=w218:dbl, element #2=w217:dbl)
    "High Velocity" <- w217
    "Low Velocity" <- w218
    n177 = Index Array(array=w224, index #1=0 ("index"), index #2=1 ("index")) -> (element #1=w216:dbl, element #2=w215:dbl)
    "High Charge Limit (fC)" <- w215
    "Low Charge Limit (fC)" <- w216
    n178 = Index Array(array=w221, index #1=0 ("index"), index #2=1 ("index")) -> (element #1=w214:dbl, element #2=w213:dbl)
    "Low Mass (kg)" <- w214
    "High Mass (kg)" <- w213
    n179 = property on="Peletron (MV)" class="DigNum (strict)"() -> ("Value"=w233:dbl)  [unwired: 2 in, 2 out]
    n180 = local read "Update Threshold"() -> (w184:bool)
    n181 = local read "Auto Threshold"() -> (w187:bool)
    n182 = Bundle("Numeric"=w218, "Numeric"=w217, "Numeric"=w216, "Numeric"=w215, "Numeric"=w214, "Numeric"=w213, w210, 26666666.6, "Value"=w233, w206, w151) -> (w275:T6)  [unwired: 1 in]
    n183 = Or(x=w187, y=w184) -> (x .or. y?=w186:bool)
    n184 = Or(x=w187, y=w189) -> (x .or. y?=w188:bool)
    n185 = call-poly <userlib>:"Data Changed__ogtk.vi"("Boolean"=w184) -> ("Changed"=w185:bool)
    n186 = case shown="True" w207 {
      frame False {
      }
      frame True {
        n187 = stacked-sequence {
          frame #0 {
            n188 = property on="Delay Ring" class="Ring (strict)"() -> ("StringsAndValues[]"=w345:T7)  [unwired: 2 in, 2 out]
            n189 = for {
              tunnel: w345 -> [w355] mode=indexing
              tunnel: [w354] -> w344 mode=indexing
              n190 = Unbundle(w355) -> ("Value"=w354:dbl)  [unwired: 1 out]
            }
            n191 = Array Size(array=w345) -> (size(s)=w348:i32)
            n192 = Decrement(x=w348) -> (x-1=w347:i32)
            n193 = Bundle("Delay Name"="Delay Name", "Delay Value"="Delay Value") -> (w350:cluster{"Delay Name":string, "Delay Value":dbl})  [unwired: 1 in]
            n194 = Insert Into Array(array=w345, index=w347, new element=w350) -> (w349:T7)
            n195 = Search 1D Array(1D array=w344, element="Delay Value") -> (index of element=w352:i32)  [unwired: 1 in]
            n196 = Equal?(x=w352, y=-1) -> (x = y?=w346:bool)
            n197 = case shown="True" w346 {
              tunnel: w349 -> [_ w364]
              frame False {
                n198 = One Button Dialog(message="Value Already Exists") -> ()  [unwired: 1 in, 1 out]
              }
              frame True {
                n199 = property on="Delay Ring" class="Ring (strict)"("StringsAndValues[]"=w364) -> ()  [unwired: 2 in, 2 out]
                n200 = Array Size(array=w364) -> (size(s)=w366:i32)
                n201 = Decrement(x=w366) -> (x-1=w365:i32)
                n202 = for {
                  N: w365 -> [_]
                  tunnel: w364 -> [w380] mode=indexing
                  tunnel: [w375] -> w367 mode=indexing
                  n203 = Unbundle(w380) -> ("String"=w376:string, "Value"=w379:dbl)
                  n204 = Format Into String(format string="%f", w379) -> (resulting string=w377:string)  [unwired: 2 in, 1 out]
                  n205 = Build Array(w376, w377) -> (w375:string[])
                }
                n206 = call <userlib>:"Current VI's Path__ogtk.vi"() -> ("Current VI's Path (+ Relative)"=w370:path)  [unwired: 1 in]
                n207 = Strip Path(path=w370) -> (stripped path=w358:path)  [unwired: 1 out]
                n208 = call-poly <userlib>:"Strip Path Extension__ogtk.vi"("path"=w358) -> ("extension"=w361:string)  [unwired: 1 out]
                n209 = Equal?(x="exe", y=w361) -> (x = y?=w359:bool)
                n210 = case shown="False" w359 {
                  tunnel: w358 -> [w372 w374]
                  tunnel: [w372 w373] -> w357
                  frame False {
                  }
                  frame True {
                    n211 = Strip Path(path=w374) -> (stripped path=w373:path)  [unwired: 1 out]
                  }
                }
                n212 = Array To Spreadsheet String(array=w367, 3:"%s" ("format string")) -> (spreadsheet string=w363:string)  [unwired: 1 in]
                n213 = Build Path(base path=w357, name or relative path="delay_ring.txt") -> (appended path=w368:path)
                n214 = call <vilib>:"Trim Whitespace.vi"("string"=w363) -> ("trimmed string"=w362:string)  [unwired: 1 in]
                n215 = Write to Text File(file (use dialog)=w368, text=w362) -> ()  [unwired: 2 in, 3 out]
              }
            }
          }
          frame #1 {
            n216 = property on="Add Delay" class="Bool (strict)"("Value"=FALSE ("Add Delay")) -> ()  [unwired: 2 in, 2 out]
          }
        }
      }
    }
    n217 = call "process_limits.vi"("old output cluster"=w282, "Input cluster"=w275) -> ("Update FPGA"=w209:bool, "output cluster"=w283:T8)  [unwired: 8 in]
    n218 = Or(x=w209, y=w188) -> (x .or. y?=w193:bool)
    n219 = And(x=w185, y=w184) -> (x .and. y?=w183:bool)
    n220 = case shown="True" w183 {
      frame False {
      }
      frame True {
        n221 = local write "Update Threshold"(FALSE ("Update Threshold")) -> ()
      }
    }
    n222 = Wait (ms)(milliseconds to wait=u32 100) -> ()  [unwired: 1 out]
    n223 = shared-variable "My Computer\\Network Shared Variables.lvlib\\FPGA Trigger"() -> ()  [unwired: 1 in, 2 out]
    n224 = Build Array("Filter1 Threshold", "Filter2 Threshold", "Filter3 Threshold", "Filter4 Threshold", "Filter5 Threshold", "Filter6 Threshold", "Filter7 Threshold") -> (w149:i32[])
    n225 = Or(x="Raise Threshold", y="Lower Threshold") -> (x .or. y?=w164:bool)
    n226 = case shown="True" "Raise Threshold" {
      tunnel: w149 -> [_ w336]
      tunnel: w150 -> [_ w326]
      frame False {
      }
      frame True {
        n227 = Subtract(x=w336, y=w326) -> (x-y=w327:i32[])
        n228 = local write "Raise Threshold"(FALSE ("Raise Threshold")) -> ()
        n229 = Index Array(array=w327) -> (element #1=w334:i32, element #2=w333:i32, element #3=w332:i32, element #4=w331:i32, element #5=w330:i32, element #6=w329:i32, element #7=w328:i32)  [unwired: 7 in]
        n230 = local write "Filter1 Threshold"(w334) -> ()
        n231 = local write "Filter2 Threshold"(w333) -> ()
        n232 = local write "Filter3 Threshold"(w332) -> ()
        n233 = local write "Filter4 Threshold"(w331) -> ()
        n234 = local write "Filter5 Threshold"(w330) -> ()
        n235 = local write "Filter6 Threshold"(w329) -> ()
        n236 = local write "Filter7 Threshold"(w328) -> ()
      }
    }
    n237 = case shown="True" "Lower Threshold" {
      tunnel: w149 -> [w314 w325]
      tunnel: w150 -> [_ w324]
      tunnel: [w314 w315] -> w178
      frame False {
      }
      frame True {
        n238 = Add(x=w325, y=w324) -> (x+y=w315:i32[])
        n239 = local write "Lower Threshold"(FALSE ("Lower Threshold")) -> ()
        n240 = Index Array(array=w315) -> (element #1=w322:i32, element #2=w321:i32, element #3=w320:i32, element #4=w319:i32, element #5=w318:i32, element #6=w317:i32, element #7=w316:i32)  [unwired: 7 in]
        n241 = local write "Filter1 Threshold"(w322) -> ()
        n242 = local write "Filter2 Threshold"(w321) -> ()
        n243 = local write "Filter3 Threshold"(w320) -> ()
        n244 = local write "Filter4 Threshold"(w319) -> ()
        n245 = local write "Filter5 Threshold"(w318) -> ()
        n246 = local write "Filter6 Threshold"(w317) -> ()
        n247 = local write "Filter7 Threshold"(w316) -> ()
      }
    }
    n248 = Or(x=w164, y=w193) -> (x .or. y?=w165:bool)
    n249 = Or(x=w165, y=w153) -> (x .or. y?=w154:bool)
    "Updating FPGA" <- w154
    n250 = Unbundle By Name(w283) -> ("Low Velocity Count"=w271:i32, "High Velocity Count"=w270:i32, "Low Charge Limit (ADC ticks)"=w268:i16, "High Charge Limit (ADC ticks)"=w269:i16, "Low Mass (ADC*cycle^2)"=w273:i64, "High Mass (ADC*cycle^2)"=w274:i64, "Mult"=w205:fxp<+,16,7>)
    "Low velocity count" <- w271
    "High velocity count" <- w270
    "High Charge Limit" <- w269
    "Low Charge Limit" <- w268
    "High Mass Limit" <- w274
    "Low Mass Limit" <- w273
    n251 = Index Array(array=w178) -> (element #1=w181:i32, element #2=w179:i32, element #3=w176:i32, element #4=w174:i32, element #5=w172:i32, element #6=w170:i32, element #7=w168:i32)  [unwired: 7 in]
    n252 = case shown="True" w154 {
      tunnel: w204 -> [w383 w411]
      tunnel: w203 -> [w384 w410]
      tunnel: [w383 w409] -> w306
      tunnel: [w384 w408] -> w305
      tunnel: w181 -> [_ w407]
      tunnel: w179 -> [_ w406]
      tunnel: w176 -> [_ w405]
      tunnel: w174 -> [_ w404]
      tunnel: w172 -> [_ w403]
      tunnel: w170 -> [_ w402]
      tunnel: w168 -> [_ w401]
      tunnel: [w382 w387] -> w280
      tunnel: w274 -> [_ w393]
      tunnel: w273 -> [_ w392]
      tunnel: w271 -> [_ w391]
      tunnel: w270 -> [_ w390]
      tunnel: w269 -> [_ w389]
      tunnel: w268 -> [_ w388]
      tunnel: w281 -> [w382 _]
      tunnel: w205 -> [_ w385]
      frame False {
      }
      frame True {
        n253 = Get Date/Time In Seconds() -> (seconds since 1Jan1904=→"Last Update:":timestamp)
        n254 = xnode "Read/Write Control"("FPGA VI Reference In"=w411, "error in"=w410, "Low Velocity Count"=w391, "High Velocity Count"=w390, "Filter threshold 1"=w407, "Filter threshold 2"=w406, "Filter threshold 3"=w405, "Filter threshold 4"=w404, "Filter threshold 5"=w403, "Filter threshold 6"=w402, "Filter threshold 7"=w401, "High Charge Limit"=w389, "Low Charge Limit"=w388, "High Mass Limit"=w393, "Low Mass Limit"=w392, "Mult1"=w385) -> ("FPGA VI Reference Out"=w409:refnum<k20>, "error out"=w408:errorcluster, "Detector 3 Correlation 1"=w400:i16, "Detector 3 Correlation 2"=w399:i16, "Detector 3 Correlation 3"=w398:i16, "Detector 3 Correlation 4"=w397:i16, "Detector 3 Correlation 5"=w396:i16, "Detector 3 Correlation 6"=w395:i16, "Detector 3 Correlation 7"=w394:i16)
        n255 = Bundle("Detector 3 Correlation 1"=w400, "Detector 3 Correlation 2"=w399, "Detector 3 Correlation 3"=w398, "Detector 3 Correlation 4"=w397, "Detector 3 Correlation 5"=w396, "Detector 3 Correlation 6"=w395, "Detector 3 Correlation 7"=w394) -> (w387:T9)  [unwired: 1 in]
      }
    }
    n256 = call "filter_peaks.vi"("Correlation cluster"=w280, "Filter peak cluster"=w276, "Zero out"="Zero Peak Values", "Run Mode"="Run Mode") -> ("Blinking"=w267:bool, "status"=w272:T2, "Filter peak output"=w277:T4)  [unwired: 5 in]
    n257 = property on="Filter 3 Peak" class="DigNum (strict)"("DisabledEnum"=w272, "Blinking"=w267) -> ()  [unwired: 2 in, 2 out]
    n258 = property on="Filter 4 Peak" class="DigNum (strict)"("DisabledEnum"=w272, "Blinking"=w267) -> ()  [unwired: 2 in, 2 out]
    n259 = property on="Filter 7 Peak" class="DigNum (strict)"("DisabledEnum"=w272, "Blinking"=w267) -> ()  [unwired: 2 in, 2 out]
    n260 = property on="Filter 5 Peak" class="DigNum (strict)"("DisabledEnum"=w272, "Blinking"=w267) -> ()  [unwired: 2 in, 2 out]
    n261 = property on="Filter 6 Peak" class="DigNum (strict)"("DisabledEnum"=w272, "Blinking"=w267) -> ()  [unwired: 2 in, 2 out]
    n262 = property on="Filter 2 Peak" class="DigNum (strict)"("DisabledEnum"=w272, "Blinking"=w267) -> ()  [unwired: 2 in, 2 out]
    n263 = property on="Filter 1 Peak" class="DigNum (strict)"("DisabledEnum"=w272, "Blinking"=w267) -> ()  [unwired: 2 in, 2 out]
    n264 = Unbundle By Name(w277) -> ("Filter 1 Peak"=w303:i32, "Filter 2 Peak"=w302:i32, "Filter 3 Peak"=w301:i32, "Filter 4 Peak"=w300:i32, "Filter 5 Peak"=w299:i32, "Filter 6 Peak"=w298:i32, "Filter 7 Peak"=w297:i32)
    "Filter 1 Peak" <- w303
    "Filter 2 Peak" <- w302
    "Filter 3 Peak" <- w301
    "Filter 4 Peak" <- w300
    "Filter 5 Peak" <- w299
    "Filter 6 Peak" <- w298
    "Filter 7 Peak" <- w297
    "Sensitivity" <- w210
  }
  n265 = while {
    stop <- w701 stop-if-true
    n266 = case shown="True" "Rate Limiting" {
      frame False {
        n267 = property on="Rearm Trigger" class="Bool (strict)"("DisabledEnum"=T2."Enabled" ("Disabled")) -> ()  [unwired: 2 in, 2 out]
        n268 = property on="One Shot Mode" class="Bool (strict)"("DisabledEnum"=T2."Enabled" ("Disabled")) -> ()  [unwired: 2 in, 2 out]
      }
      frame True {
        n269 = local read "Armed"() -> (w705:bool)
        n270 = Get Date/Time In Seconds() -> (seconds since 1Jan1904=w704:timestamp)
        n271 = property on="Rearm Trigger" class="Bool (strict)"("DisabledEnum"=T2."Disabled and Grayed Out" ("Disabled")) -> ()  [unwired: 2 in, 2 out]
        n272 = case shown="False" w705 {
          tunnel: [w712 FALSE] -> w709
          tunnel: w704 -> [w711 _]
          frame False {
            n273 = flat-sequence {
              tunnel: w711 -> [w713]
              tunnel: [w713] -> w710
              tunnel: [TRUE] -> w712
              tunnel: w710 -> [w719]
              frame #0 {
                n274 = Multiply(x="Min. Time\nBetween Shots (s)", y=1000.0) -> (x*y=w716:dbl)
                n275 = Round Toward +Infinity(x=w716) -> (ceil(x): smallest int >= x=w714:dbl)
                n276 = Wait (ms)(milliseconds to wait=w714) -> ()  [unwired: 1 out]
              }
              frame #1 {
                n277 = Get Date/Time In Seconds() -> (seconds since 1Jan1904=w720:timestamp)
                n278 = Subtract(x=w720, y=w719) -> (x-y=→"Time Betwee Shots":dbl)
              }
            }
          }
          frame True {
          }
        }
        n279 = property on="One Shot Mode" class="Bool (strict)"("DisabledEnum"=T2."Disabled and Grayed Out" ("Disabled"), "Value"=TRUE ("One Shot Mode")) -> ()  [unwired: 2 in, 2 out]
        n280 = local write "Rearm Trigger"(w709) -> ()
      }
    }
    n281 = property on="stopping" class="Bool (strict)"() -> ("Value"=w701:bool)  [unwired: 2 in, 2 out]
  }
  n282 = call "connect out.vi"("error in (no error)"=w15, "connection reference"=w17) -> ()  [unwired: 9 in, 1 out]
  n283 = xnode "Close FPGA VI Reference"("FPGA VI Reference In"=w41, "error in"=w40) -> ("error out"=w43:errorcluster)
  n284 = call <vilib>:"General Error Handler.vi"("error in (no error)"=w43) -> ()  [unwired: 10 in, 5 out]
